vi "Evaluation.vi"(6 "ToEvaluate in":refnum<data-value>, 8 "error in (no error)":errorcluster, 10 "Parents G":dbl, 11 "PathTree in":refnum<class "RouteTree.lvclass">) -> (0 "error out":errorcluster, 1 "H":dbl, 2 "G":dbl, 3 "PathTree out":refnum<class "RouteTree.lvclass">, 4 "ToEvaluate out":refnum<data-value>)   [LabVIEW 2014, in "RouteTree.lvclass"]
uses:
  <userlib>/AdvancedDataStructures/ClassBased/Applications/RouteSearch/PathTree/RouteTree.lvclass
  <userlib>/AdvancedDataStructures/ClassBased/TreeNode/TreeNode.lvclass
  <userlib>/AdvancedDataStructures/ClassBased/Applications/RouteSearch/Waypoint/Waypoint.lvclass
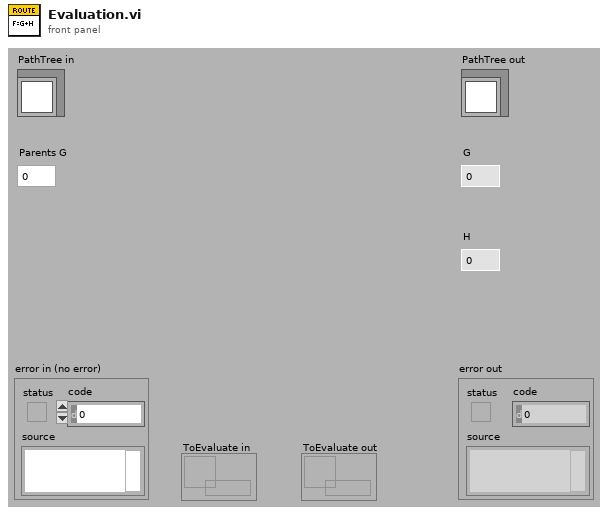
[diagram p1: front panel]
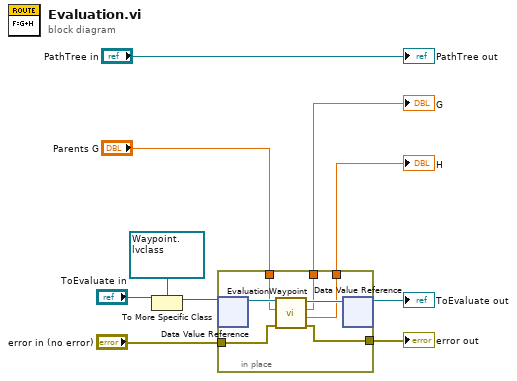
[diagram p0: block diagram]
diagram:
  n1 = To More Specific Class(target class=refnum<data-value> refnum ("data value reference"), reference="ToEvaluate in") -> (specific class reference=w7:refnum<data-value>)  [unwired: 1 in, 1 out]
  n2 = in-place {
    in-place-border: "Parents G" -> [w16]
    in-place-border: "error in (no error)" -> [w15]
    in-place-border: [w14] -> w1
    in-place-border: [w12] -> w3
    in-place-border: [w11] -> w2
    n3 = in-place-dvr #1(w7) -> (w17:refnum<class "Waypoint.lvclass">)  [unwired: 1 out]
    n4 = call <userlib>:"EvaluationWaypoint.vi"("error in (no error)"=w15, "Parents G"=w16, "Waypoint in"=w17) -> ("error out"=w14:errorcluster, "H"=w11:dbl, "G"=w12:dbl, "Waypoint out"=w13:refnum<class "Waypoint.lvclass">)  [unwired: 5 in]
    n5 = in-place-dvr #1(w13) -> (→"ToEvaluate out":refnum<data-value>)  [unwired: 1 out]
  }
  "error out" <- w1
  "G" <- w3
  "H" <- w2
  "PathTree out" <- "PathTree in"
